vi "BLDCMotor Example.vi"() -> ()   [LabVIEW 2012, in "Phidget BLDC Motor.lvlib"]
uses:
  <instrlib>/Phidgets/Phidget BLDC Motor/Phidget BLDC Motor.lvlib
  <instrlib>/Phidgets/Phidget BLDC Motor/Public/BLDCMotorStart.vi
  <instrlib>/Phidgets/Phidget BLDC Motor/Public/BLDCMotorClose.vi
  <instrlib>/Phidgets/Phidget Common/Phidget Common.lvlib
panel:
  in  "Velocity":dbl(slide) caption="Duty Cycle" scale=-1.0..1.0
  in  "Stall Velocity":dbl=1000.0
  in  "Acceleration":dbl=1.0
  in  "stop":bool
  in  "Device Info":T1={"Serial Number"=-1, "Channel"=0, "Port"=0}
  out "Attached?":bool
  out "Serial Number Return":i32
  out "error out":errorcluster
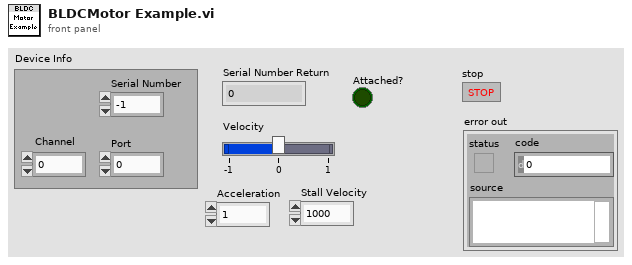
[diagram p1: front panel]
types:
  T1 = cluster{"Serial Number":i32, "Channel":i32, "Port":i32}
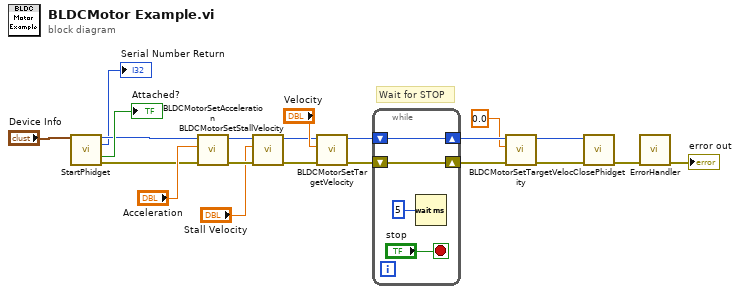
[diagram p0: block diagram]
diagram:
  # "Wait for STOP"
  n1 = call-poly <instrlib>:"StartPhidget.vi"("Device Info"="Device Info") -> ("Phidget ID"=w17:u64, "Serial Number Return"=→"Serial Number Return":i32, "Attached?"=→"Attached?":bool, "error out"=w10:errorcluster)  [unwired: 11 in]
  n2 = call <instrlib>:"BLDCMotorSetAcceleration.vi"("error in (no error)"=w10, "Acceleration"="Acceleration", "Device In"=w17) -> ("error out"=w8:errorcluster, "Device Out"=w7:u64)  [unwired: 6 in]
  n3 = call <instrlib>:"BLDCMotorSetStallVelocity.vi"("error in (no error)"=w8, "Stall Velocity"="Stall Velocity", "Device In"=w7) -> ("error out"=w3:errorcluster, "Device Out"=w4:u64)  [unwired: 6 in]
  n4 = call <instrlib>:"BLDCMotorSetTargetVelocity.vi"("error in (no error)"=w3, "Velocity"="Velocity", "Device In"=w4) -> ("error out"=w1:errorcluster, "Device Out"=w2:u64)  [unwired: 6 in]
  n5 = while {
    shift-right: [w22] -> w16
    shift-left: w2 -> [w22]
    shift-right: [w23] -> w15
    shift-left: w1 -> [w23]
    stop <- "stop" stop-if-true
    n6 = Wait (ms)(milliseconds to wait=u32 5) -> ()  [unwired: 1 out]
  }
  n7 = call <instrlib>:"BLDCMotorSetTargetVelocity.vi"("error in (no error)"=w15, "Velocity"=0.0 ("Velocity Limit"), "Device In"=w16) -> ("error out"=w14:errorcluster, "Device Out"=w13:u64)  [unwired: 6 in]
  n8 = call-poly <instrlib>:"ClosePhidget.vi"("error in"=w14, "Device In"=w13) -> ("error out"=w21:errorcluster)  [unwired: 9 in]
  n9 = call <instrlib>:"ErrorHandler.vi"("error in"=w21) -> ("error out"=→"error out":errorcluster)  [unwired: 9 in, 1 out]
